vi "AMX-CCD3 自动处理图像.vi"(5 "All Files in Dir 2":path[](array[path]), 7 "数值 2":i32, 9 "A/B段位置切换":bool, 11 "error in (no error)":errorcluster caption="错误输入（无错误）") -> (3 "处理时间":dbl, 4 "Image Out":T1(plugin-control), 6 "结果":bool, 8 "数值 3":i32, 10 "颗粒物有无判断":bool, 14 "结果数组":bool[](array[boolean]), 15 "error out":errorcluster caption="错误输出")   [LabVIEW 2017]
uses:
  Global System.vi
panel:
  out "路径":path
  out "x = y?":bool[](array[boolean])
  out "处理完成文件":string[](array[string])
  out "子字符串":string
  out "未处理文件":string[](array[string])
  in  "颗粒物个数阈值":i32
  out "单个图片路径":path
  out "颗粒物大小显示":dbl[](array[numeric])
  out "颗粒物位置坐标":cluster{"X":dbl, "Y":dbl}[](array[cluster]) {"Y" format="%.2f"; "X" format="%.2f"}
  out "All Files in Dir":path[](array[path]) caption="目录中的所有文件"
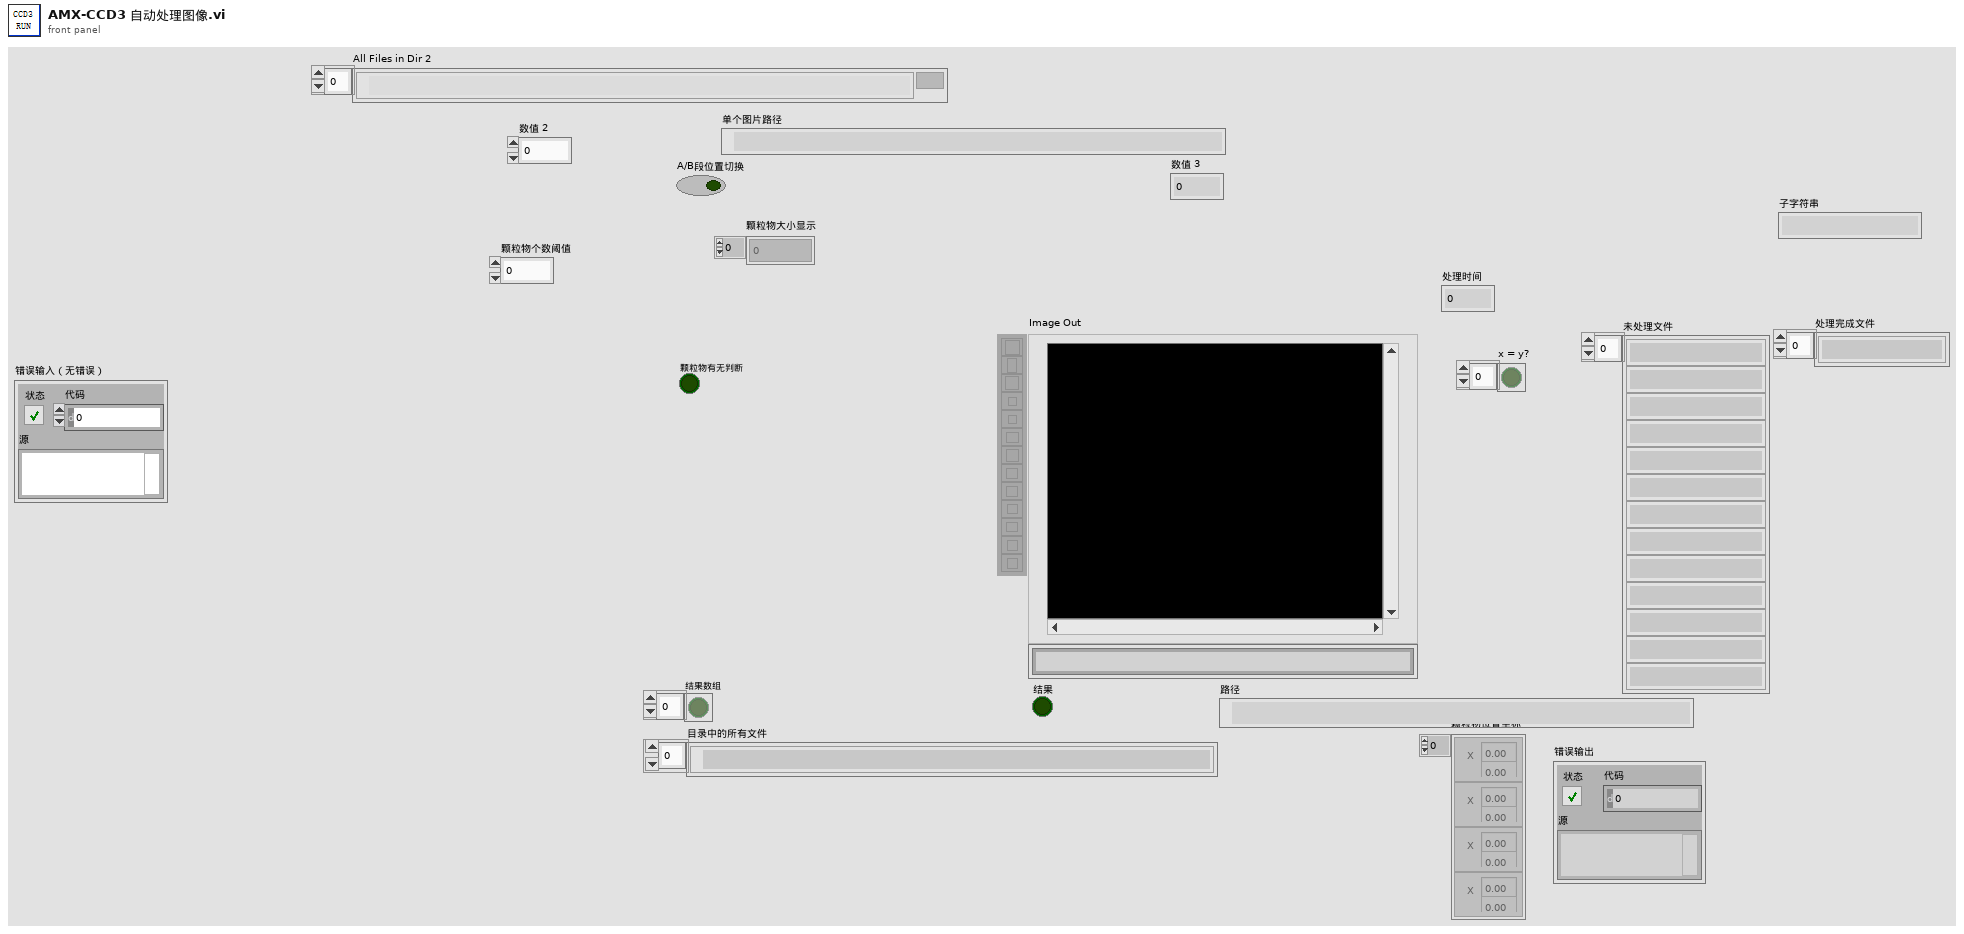
[diagram p1: front panel]
types:
  T1 = typedef "IMAQ Image.ctl" = refnum<image>
  T2 = typedef "Image Type" = u32
  T3 = typedef "IMAQ Rectangle" = cluster{"Left":i32, "Top":i32, "Right":i32, "Bottom":i32, "Rotation":dbl}
  T4 = cluster{"Rectangle":T3, "Threshold Limits (Threshold 1)":cluster{"Lower value":sgl, "Upper value":sgl}, "Keep/Remove Particles ":bool, "Connectivity 4/8 (8) ":bool, "Selection Values (Particle Filter 1)":cluster{"Measurement Parameter":i32, "Range Lower Value":dbl, "Range Upper Value":dbl, "Range":bool, "Measurement Type":bool}[], "Corner Options (Feature Detection 1)":cluster{"Detector type":enum32{"Harris Corner", "Shi-Tomasi Corner"}, "Kernel size":i32, "Min Corner Point Strength":dbl}, "Pyramid level (Feature Detection 1)":u32, "Method ":i32, "Look For":u32, "Method 2":i32, "ROI Descriptor (Clamp (Rake) 1)":cluster{"Global Rectangle":i32[], "Contours":cluster{"ID":enum32{"External", "Internal"}, "Type":u32, "Coordinates":i32[]}[]}}
  T5 = typedef "IMAQ Curve Parameters.ctl" = cluster{"Extraction Mode":u32, "Edge Threshold":i32, "Edge Filter Size":u32, "Min Length":i32, "Row Search Step Size":i32, "Col Search Step Size":i32, "Max Endpoint Gap":i32, "Closed":bool, "Subpixel":bool}
  T6 = cluster{"Curve Extraction Settings ":T5, "Color Mode (Histogram 1)":u16, "Range (Threshold 1)":cluster{"Lower value":sgl, "Upper value":sgl}, "Clamp Settings (Max Clamp 1)":cluster{"Angle Range (+/-)":dbl, "Edge Polarity":cluster{"Start":u32, "End":u32}}, "Settings (Clamp (Rake) 1)":cluster{"Contrast":i32, "Filter width":i32, "Steepness":i32, "Subsampling Ratio":u32, "Show Search Area":bool, "Show Search Lines":bool, "Show Edges Found":bool, "Show Result":bool}, "直径设定":cluster{"Lower value":sgl, "Upper value":sgl}}
  T7 = typedef "IMAQdx.ctl" = refnum<k21>
  T8 = cluster{"IsNorImage":bool, "Exposure Values":u32, "ImagePath":path, "相机选择":T7}
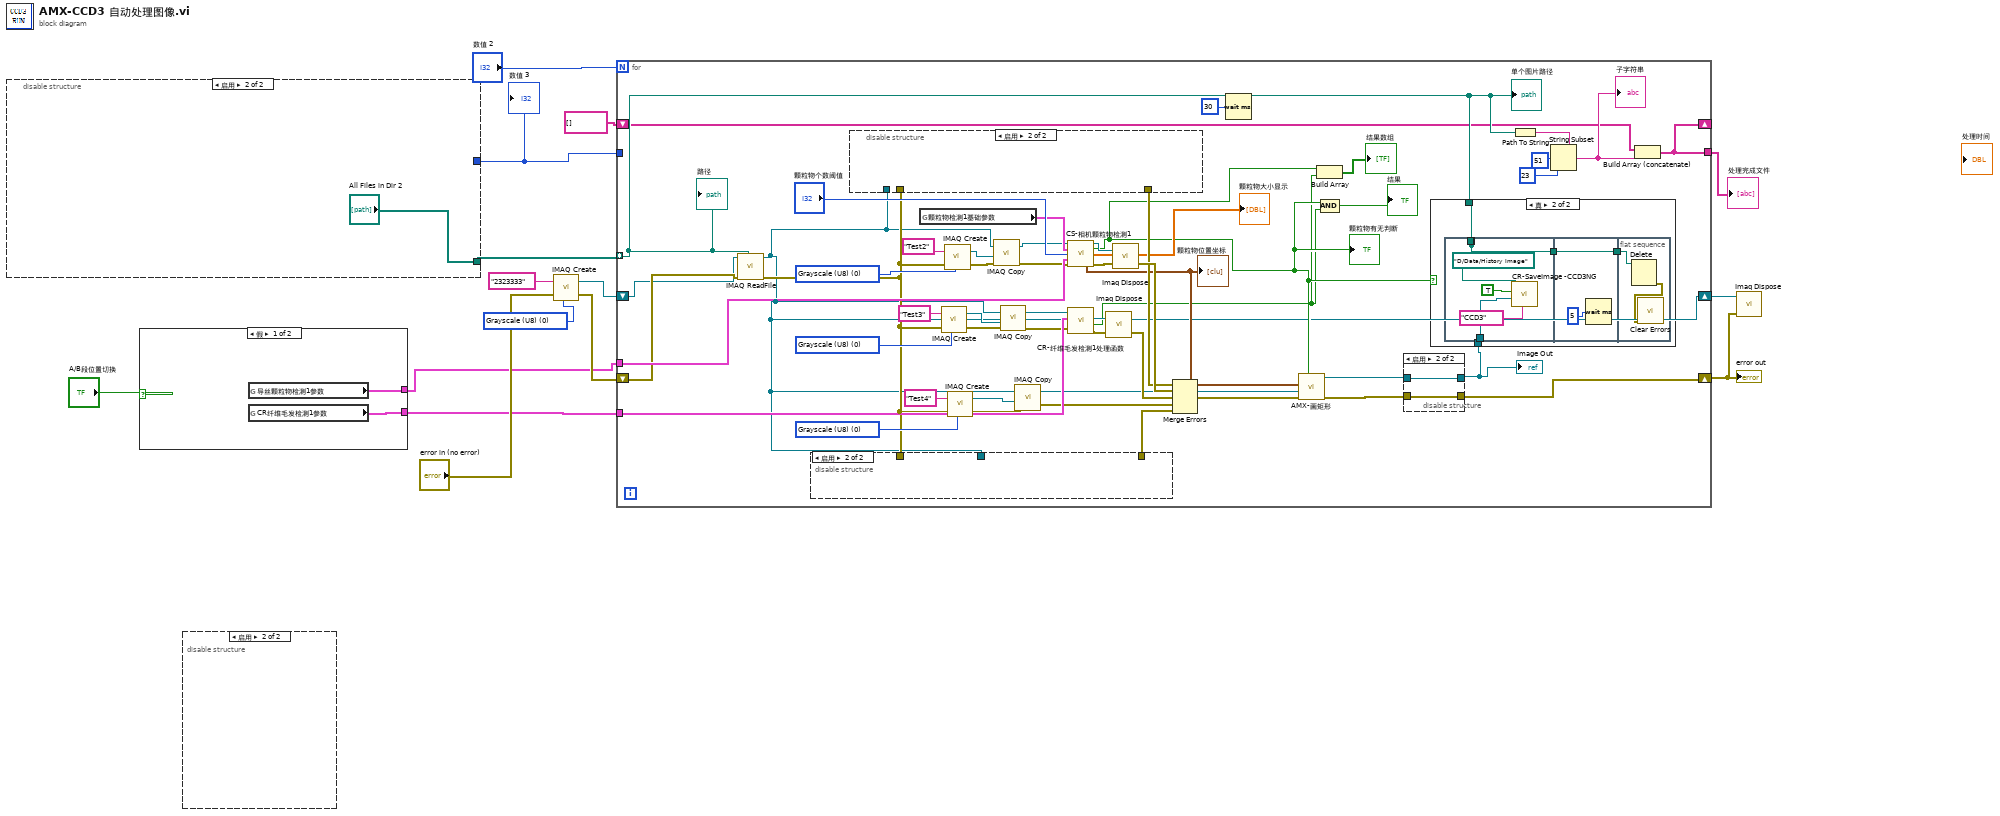
[diagram p0: block diagram]
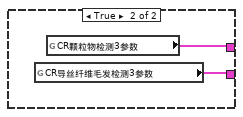
[diagram p2: hidden frame]
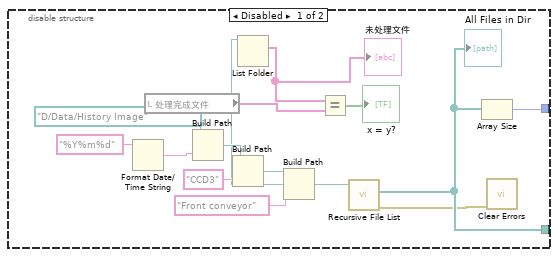
[diagram p3: hidden frame]
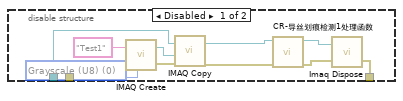
[diagram p4: hidden frame]
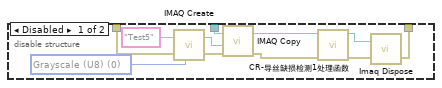
[diagram p5: hidden frame]
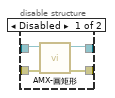
[diagram p6: hidden frame]
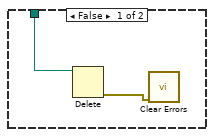
[diagram p7: hidden frame]
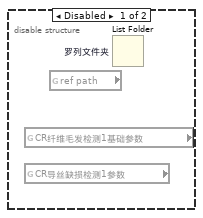
[diagram p8: hidden frame]
diagram:
  w8 = T2 0 items=["Grayscale (U8)", "Grayscale (I16)", "Grayscale (SGL)", "Complex (CSG)", "RGB (U32)", "HSL (U32)", "RGB (U64)", "Grayscale (U16)"] ("Image Type")
  n1 = disable-structure shown="启用" {
    disable-tunnel: [w22 _] -> w15
    disable-tunnel: [w21 "All Files in Dir 2"] -> w14
    frame Disabled {
      n2 = Format Date/Time String(time format string (%c)="%Y%m%d" ("时间格式字符串(%c)")) -> (date/time string=w23:string)  [unwired: 2 in]
      n3 = local read "处理完成文件"() -> (w18:string[])
      n4 = Build Path(base path=path "D:/Data/History Image" ("基路径"), name or relative path=w23) -> (appended path=w26:path)
      n5 = Build Path(base path=w26, name or relative path="CCD3" ("名称或相对路径")) -> (appended path=w24:path)
      n6 = Build Path(base path=w24, name or relative path="Front conveyor" ("名称或相对路径")) -> (appended path=w20:path)
      n7 = List Folder(path=w20) -> (filenames=w19:string[])  [unwired: 3 in, 3 out]
      "未处理文件" <- w19
      n8 = Equal?(x=w19, y=w18) -> (x = y?=→"x = y?":bool[])
      n9 = call <vilib>:"Recursive File List.vi"("Folder Path"=w20) -> ("error out"=w16:errorcluster, "All Files in Dir"=w21:path[])  [unwired: 6 in, 3 out]
      "All Files in Dir" <- w21
      n10 = Array Size(array=w21) -> (size(s)=w22:i32)
      n11 = call <vilib>:"Clear Errors.vi"("error in (no error)"=w16) -> ()  [unwired: 5 in, 2 out]
    }
    frame Enabled {
    }
  }
  "数值 3" <- w15
  n12 = case shown="假" "A/B段位置切换" {
    tunnel: [w32 w34] -> w2
    tunnel: [w31 w33] -> w1
    frame False {
      n13 = global read "Global System.vi" "导丝颗粒物检测1参数"() -> (w32:T4)
      n14 = global read "Global System.vi" "CR纤维毛发检测1参数"() -> (w31:T6)
    }
    frame True {
      n15 = global read "Global System.vi" "CR导丝纤维毛发检测3参数"() -> (w33:T6)
      n16 = global read "Global System.vi" "CR颗粒物检测3参数"() -> (w34:T4)
    }
  }
  n17 = disable-structure shown="启用" {
    frame Disabled {
      n18 = global read "Global System.vi" "CR纤维毛发检测1基础参数"() -> ()  [unwired: 1 out]
      n19 = global read "Global System.vi" "CR导丝缺损检测1参数"() -> ()  [unwired: 1 out]
      n20 = global read "Global System.vi" "ref path"() -> ()  [unwired: 1 out]
      n21 = List Folder "罗列文件夹"() -> ()  [unwired: 4 in, 4 out]
    }
    frame Enabled {
    }
  }
  n22 = call "IMAQ Create"("Image Name"="2323333", "Image Type"=w8, "error in (no error)"="error in (no error)") -> ("New Image"=w5:T1, "error out"=w6:errorcluster)  [unwired: 2 in]
  n23 = for {
    N: "数值 2" -> [_]
    tunnel: w14 -> [w62] mode=indexing
    shift-right: [w87] -> w3
    shift-left: w6 -> [w37]
    tunnel: w15 -> [_]
    shift-right: [w56] -> _
    shift-left: string[] [] ("添加的数组") -> [w57]
    tunnel: [w56] -> w12
    tunnel: w1 -> [w55]
    tunnel: w2 -> [w54]
    shift-right: [w35] -> w4
    shift-left: w5 -> [w36]
    w69 = T2 0 items=["Grayscale (U8)", "Grayscale (I16)", "Grayscale (SGL)", "Complex (CSG)", "RGB (U32)", "HSL (U32)", "RGB (U64)", "Grayscale (U16)"] ("Image Type")
    w71 = T2 0 items=["Grayscale (U8)", "Grayscale (I16)", "Grayscale (SGL)", "Complex (CSG)", "RGB (U32)", "HSL (U32)", "RGB (U64)", "Grayscale (U16)"] ("Image Type")
    w76 = T2 0 items=["Grayscale (U8)", "Grayscale (I16)", "Grayscale (SGL)", "Complex (CSG)", "RGB (U32)", "HSL (U32)", "RGB (U64)", "Grayscale (U16)"] ("Image Type")
    n24 = call "IMAQ ReadFile"("File Path"=w62, "error in (no error)"=w37, "Image"=w36) -> ("error out"=w38:errorcluster, "Image Out"=w35:T1)  [unwired: 4 in, 3 out]
    n25 = disable-structure shown="启用" {
      disable-tunnel: [w109 _] -> w83
      disable-tunnel: w38 -> [w103 _]
      disable-tunnel: w35 -> [w102 _]
      frame Disabled {
        w107 = T2 0 items=["Grayscale (U8)", "Grayscale (I16)", "Grayscale (SGL)", "Complex (CSG)", "RGB (U32)", "HSL (U32)", "RGB (U64)", "Grayscale (U16)"] ("Image Type")
        n26 = call "IMAQ Create"("Image Name"="Test5", "Image Type"=w107, "error in (no error)"=w103) -> ("New Image"=w106:T1, "error out"=w105:errorcluster)  [unwired: 2 in]
        n27 = call "IMAQ Copy"("error in (no error)"=w105, "Image Dst"=w106, "Image Src"=w102) -> ("error out"=w101:errorcluster, "Image Dst Out"=w104:T1)  [unwired: 3 in]
        n28 = call "CR-导丝缺损检测1处理函数.vi"("error in (no error)"=w101, "Image in"=w104) -> ("error out"=w99:errorcluster, "Image out"=w100:T1)  [unwired: 6 in, 2 out]
        n29 = call "Imaq Dispose"("Image"=w100, "error in (no error)"=w99) -> ("error out"=w109:errorcluster)  [unwired: 4 in]
      }
      frame Enabled {
      }
    }
    n30 = disable-structure shown="启用" {
      disable-tunnel: [w98 _] -> w80
      disable-tunnel: w38 -> [w92 _]
      disable-tunnel: w35 -> [w91 _]
      frame Disabled {
        w97 = T2 0 items=["Grayscale (U8)", "Grayscale (I16)", "Grayscale (SGL)", "Complex (CSG)", "RGB (U32)", "HSL (U32)", "RGB (U64)", "Grayscale (U16)"] ("Image Type")
        n31 = call "IMAQ Create"("Image Name"="Test1", "Image Type"=w97, "error in (no error)"=w92) -> ("New Image"=w94:T1, "error out"=w95:errorcluster)  [unwired: 2 in]
        n32 = call "IMAQ Copy"("error in (no error)"=w95, "Image Dst"=w94, "Image Src"=w91) -> ("error out"=w90:errorcluster, "Image Dst Out"=w96:T1)  [unwired: 3 in]
        n33 = call "CR-导丝划痕检测1处理函数.vi"("error in (no error)"=w90, "Image in"=w96) -> ("error out"=w88:errorcluster, "Image out"=w89:T1)  [unwired: 6 in, 2 out]
        n34 = call "Imaq Dispose"("Image"=w89, "error in (no error)"=w88) -> ("error out"=w98:errorcluster)  [unwired: 4 in]
      }
      frame Enabled {
      }
    }
    n35 = global read "Global System.vi" "颗粒物检测1基础参数"() -> (w52:T8)
    n36 = call "IMAQ Create"("Image Name"="Test3", "Image Type"=w69, "error in (no error)"=w38) -> ("New Image"=w43:T1, "error out"=w46:errorcluster)  [unwired: 2 in]
    n37 = call "IMAQ Create"("Image Name"="Test2", "Image Type"=w76, "error in (no error)"=w38) -> ("New Image"=w50:T1, "error out"=w48:errorcluster)  [unwired: 2 in]
    n38 = call "IMAQ Create"("Image Name"="Test4", "Image Type"=w71, "error in (no error)"=w38) -> ("New Image"=w42:T1, "error out"=w39:errorcluster)  [unwired: 2 in]
    n39 = call "IMAQ Copy"("error in (no error)"=w48, "Image Dst"=w50, "Image Src"=w35) -> ("error out"=w47:errorcluster, "Image Dst Out"=w49:T1)  [unwired: 3 in]
    n40 = call "IMAQ Copy"("error in (no error)"=w46, "Image Dst"=w43, "Image Src"=w35) -> ("error out"=w45:errorcluster, "Image Dst Out"=w44:T1)  [unwired: 3 in]
    n41 = call "IMAQ Copy"("error in (no error)"=w39, "Image Dst"=w42, "Image Src"=w35) -> ("error out"=w40:errorcluster, "Image Dst Out"=w41:T1)  [unwired: 3 in]
    n42 = call "CS-相机颗粒物检测1.vi"("Image in"=w49, "相机颗粒物检测1基础参数"=w52, "颗粒物个数阈值"="颗粒物个数阈值", "导丝颗粒物检测1参数"=w54, "error in (no error)"=w47) -> ("颗粒物位置坐标"=w78:cluster{"X":dbl, "Y":dbl}[], "Image out"=w75:T1, "颗粒物有无显示"=w65:bool, "颗粒物大小显示"=→"颗粒物大小显示":dbl[], "error out"=w74:errorcluster)  [unwired: 4 in, 2 out]
    "颗粒物有无判断" <- w65
    "颗粒物位置坐标" <- w78
    n43 = call "CR-纤维毛发检测1处理函数.vi"("error in (no error)"=w45, "UI电源线正面漏线参数"=w55, "Image in"=w44) -> ("error out"=w67:errorcluster, "纤维毛发"=w63:bool, "Image out"=w68:T1)  [unwired: 4 in, 2 out]
    n44 = call "Imaq Dispose"("Image"=w68, "error in (no error)"=w67) -> ("error out"=w82:errorcluster)  [unwired: 4 in]
    n45 = call "Imaq Dispose"("Image"=w75, "error in (no error)"=w74) -> ("error out"=w81:errorcluster)  [unwired: 4 in]
    n46 = Merge Errors(w80, w81, w82, w40, w83) -> (w79:errorcluster)
    n47 = Wait (ms)(milliseconds to wait=u32 30 ("等待时间（毫秒）")) -> ()  [unwired: 1 out]
    n48 = call "AMX-画矩形.vi"("布尔"=w65, "error in (no error)"=w79, "颗粒物位置坐标"=w78, "Image In"=w41) -> ("error out"=w85:errorcluster, "Image Out"=w86:T1)  [unwired: 6 in]
    n49 = Build Array(w65, w63) -> (→"结果数组":bool[])
    n50 = Compound Arithmetic op=AND ("复合运算")(w65, w63) -> (→"结果":bool)
    n51 = disable-structure shown="启用" {
      disable-tunnel: [w113 w114] -> w87
      disable-tunnel: w86 -> [w112 w115]
      disable-tunnel: w85 -> [w111 w114]
      disable-tunnel: [w110 w115] -> w53
      frame Disabled {
        n52 = call "AMX-画矩形.vi"("error in (no error)"=w111, "Image In"=w112) -> ("error out"=w113:errorcluster, "Image Out"=w110:T1)  [unwired: 8 in]
      }
      frame Enabled {
      }
    }
    "Image Out" <- w53
    n53 = case shown="真" w65 {
      tunnel: w62 -> [w117 w120]
      tunnel: w53 -> [_ w121]
      frame False {
        n54 = Delete(path (use dialog)=w117) -> (error out=w116:errorcluster)  [unwired: 4 in, 2 out]
        n55 = call <vilib>:"Clear Errors.vi"("error in (no error)"=w116) -> ()  [unwired: 5 in, 2 out]
      }
      frame True {
        n56 = flat-sequence {
          tunnel: w121 -> [w126]
          tunnel: [w122] -> _
          tunnel: w120 -> [w122]
          tunnel: [w122] -> w119
          tunnel: w119 -> [w127]
          tunnel: [w127] -> w118
          tunnel: w118 -> [w130]
          frame #0 {
            n57 = call "CR-SaveImage -CCD3NG.vi"("CCD Name"="CCD3", "Image in"=w126, "布尔"=TRUE, "基路径"=path "D:/Data/History Image") -> ()  [unwired: 7 in, 1 out]
          }
          frame #1 {
            n58 = Wait (ms)(milliseconds to wait=u32 5 ("等待时间（毫秒）")) -> ()  [unwired: 1 out]
          }
          frame #2 {
            n59 = Delete(path (use dialog)=w130) -> (error out=w129:errorcluster)  [unwired: 4 in, 2 out]
            n60 = call <vilib>:"Clear Errors.vi"("error in (no error)"=w129) -> ()  [unwired: 5 in, 2 out]
          }
        }
      }
    }
    n61 = Path To String(path=w62) -> (string=w61:string)
    n62 = String Subset(string=w61, offset (0)=51 ("偏移量(0)"), length (rest)=23 ("长度（剩余）")) -> (substring=w58:string)
    "子字符串" <- w58
    n63 = Build Array (concatenate)(w57, w58) -> (w56:string[])
    "单个图片路径" <- w62
    "路径" <- w62
  }
  "error out" <- w3
  "处理完成文件" <- w12
  n64 = call "Imaq Dispose"("Image"=w4, "error in (no error)"=w3) -> ()  [unwired: 4 in, 1 out]
